vi "setAttribute.vi"(8 "error in (no error)":errorcluster, 10 "attribute":T1, 11 "xmlNode.lvclass in":refnum<class "xmlNode.lvclass">) -> (0 "error out":errorcluster, 3 "xmlNode.lvclass out":refnum<class "xmlNode.lvclass">)   [LabVIEW 2011, in "Tools.lvlib" / "xml.lvlib" / "xmlNode.lvclass"]
doc: "Please use set all attributes instead."
uses:
  xmlNode.lvclass
  xmlNode.lvclass/xmlNode.ctl
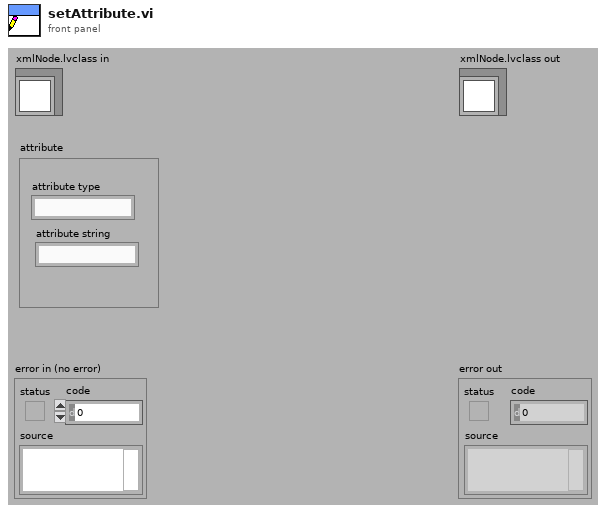
[diagram p1: front panel]
types:
  T1 = cluster{"attribute type":string, "attribute string":string}
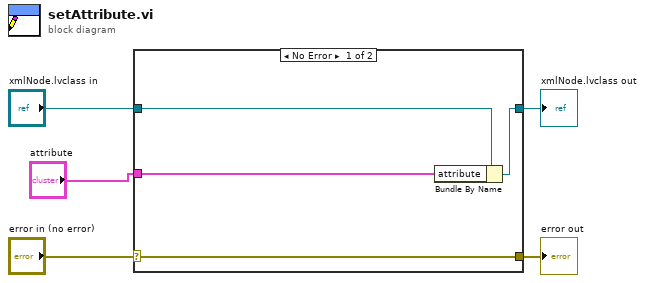
[diagram p0: block diagram]
diagram:
  n1 = case shown="No Error" "error in (no error)" {
    selector: "error in (no error)" -> [w9 w10]
    tunnel: [w9 w10] -> w4
    tunnel: [w8 w11] -> w2
    tunnel: "xmlNode.lvclass in" -> [w6 w11]
    tunnel: "attribute" -> [w7 _]
    frame No Error {
      n2 = Bundle By Name(cluster=w6, "attribute"=w7) -> (w8:refnum<class "xmlNode.lvclass">)
    }
    frame Error {
    }
  }
  "error out" <- w4
  "xmlNode.lvclass out" <- w2
